vi "GetOffsetRWIcon.vi"(6 "Whitespace color":u32(colorbox), 9 "R/W overlay":T1, 11 "Icon":T1) -> (3 "RW glyph":picture)   [LabVIEW 2020]
uses:
  <vilib>/picture/picture.llb/imagedata.ctl
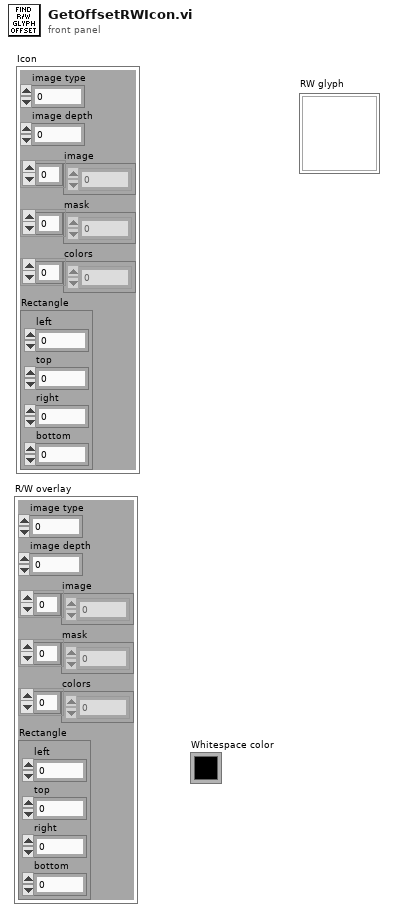
[diagram p1: front panel]
types:
  T1 = typedef "imagedata.ctl" = cluster{"image type":i32, "image depth":i32, "image":u8[], "mask":u8[], "colors":u32[], "Rectangle":cluster{"left":i16, "top":i16, "right":i16, "bottom":i16}}
  T2 = cluster{"left":i16, "top":i16, "right":i16, "bottom":i16}
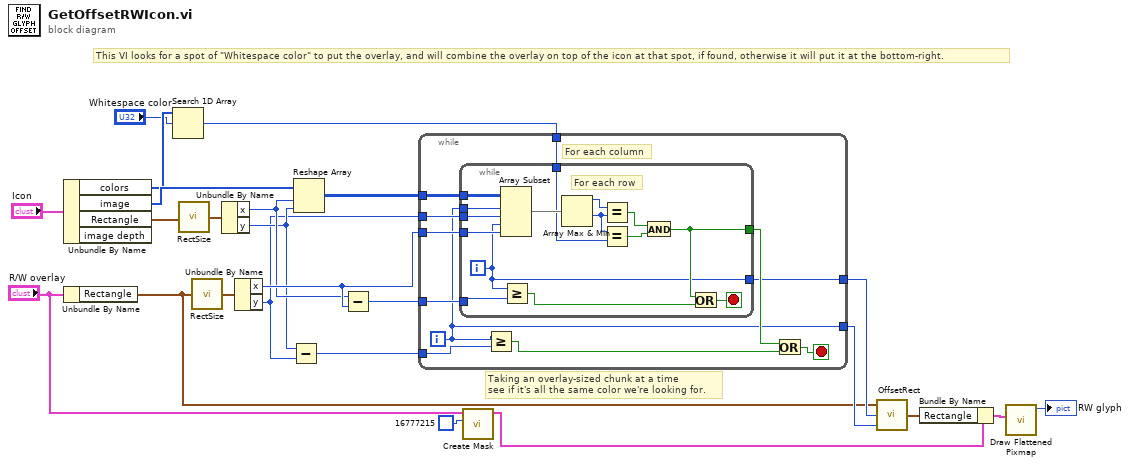
[diagram p0: block diagram]
diagram:
  # "This VI looks for a spot of \"Whitespace color\" to put the overlay, and will combine the overlay on top of the icon at that spot, if found, otherwise it will put it at the bottom-right."
  # "Taking an overlay-sized chunk at a time\nsee if it's all the same color we're looking for."
  n1 = Unbundle By Name("Icon") -> ("colors"=w14:u32[], "image"=w16:u8[], "Rectangle"=w7:T2)  [unwired: 1 out]
  n2 = Unbundle By Name("R/W overlay") -> ("Rectangle"=w9:T2)
  n3 = Search 1D Array(1D array=w14, element="Whitespace color") -> (index of element=w12:i32)  [unwired: 1 out]
  n4 = call <vilib>:"RectSize.vi"("rect"=w7) -> ("point"=w19:cluster{"x":i16, "y":i16})
  n5 = call <vilib>:"RectSize.vi"("rect"=w9) -> ("point"=w21:cluster{"x":i16, "y":i16})
  n6 = Unbundle By Name(w19) -> ("x"=w18:i16, "y"=w17:i16)
  n7 = Unbundle By Name(w21) -> ("x"=w20:i16, "y"=w15:i16)
  n8 = Subtract(x=w17, y=w15) -> (x-y=w22:i16)
  n9 = Reshape Array(w16, w18, w17) -> (w24:u8[][])
  n10 = Subtract(x=w18, y=w20) -> (x-y=w23:i16)
  n11 = while {
    tunnel: w24 -> [w35]
    tunnel: w23 -> [w31]
    tunnel: w15 -> [w30]
    tunnel: w20 -> [w34]
    tunnel: w22 -> [w32]
    tunnel: [w27] -> w11
    tunnel: [w26] -> w10
    tunnel: w12 -> [w25]
    i -> [w26]
    stop <- w33 stop-if-true
    # "For each column"
    n12 = while {
      tunnel: w35 -> [w40]
      tunnel: w30 -> [w44]
      tunnel: w34 -> [w43]
      tunnel: w31 -> [w47]
      tunnel: [w45] -> w28
      tunnel: [w41] -> w27
      tunnel: w26 -> [w42]
      tunnel: w25 -> [w36]
      i -> [w41]
      stop <- w48 stop-if-true
      # "For each row"
      n13 = Array Subset(array=w40, index (row)=w42, length (row)=w44, index (col)=w41, length (col)=w43) -> (w39:u8[][])
      n14 = Greater Or Equal?(x=w41, y=w47) -> (x >= y?=w46:bool)
      n15 = Array Max & Min(array=w39) -> (max value=w38:u8, min value=w37:u8)  [unwired: 2 out]
      n16 = Equal?(x=w38, y=w37) -> (x = y?=w50:bool)
      n17 = Equal?(x=w37, y=w36) -> (x = y?=w49:bool)
      n18 = And(x=w50, y=w49) -> (x .and. y?=w45:bool)
      n19 = Or(x=w45, y=w46) -> (x .or. y?=w48:bool)
    }
    n20 = Greater Or Equal?(x=w26, y=w32) -> (x >= y?=w29:bool)
    n21 = Or(x=w28, y=w29) -> (x .or. y?=w33:bool)
  }
  n22 = call <vilib>:"Create Mask.vi"("Mask Color (Black)"=u32 16777215, "image data"="R/W overlay") -> ("image data"=w4:T1)  [unwired: 2 in, 7 out]
  n23 = call <vilib>:"OffsetRect.vi"("v"=w10, "h"=w11, "rect"=w9) -> ("offset rect"=w8:T2)
  n24 = Bundle By Name(cluster=w4, "Rectangle"=w8) -> (w2:T1)
  n25 = call <vilib>:"Draw Flattened Pixmap.vi"("image data"=w2) -> ("new picture"=→"RW glyph":picture)  [unwired: 8 in]
